vi "EXAMEND_13_02_25.vi"() -> ()   [LabVIEW 2025]
uses:
  <vilib>/numeric/Random Number (Range) I64.vi
  <vilib>/numeric/sub_Random U32.vi
panel:
  out "ESTADO DE LA SEÑAL":string
  out "ON/OFF":bool
  out "EN RANGO":bool
  out "VALOR PERILLA":dbl
  in  "Knob":dbl(knob) scale=0.0..100.0
  out "Valor Actual":dbl
  in  "stop":bool
  out "Waveform Chart":dynamicdata(graph)
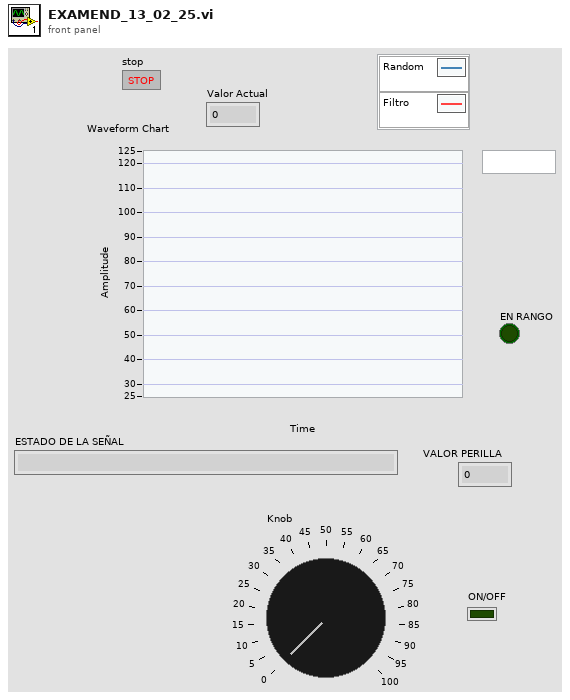
[diagram p1: front panel]
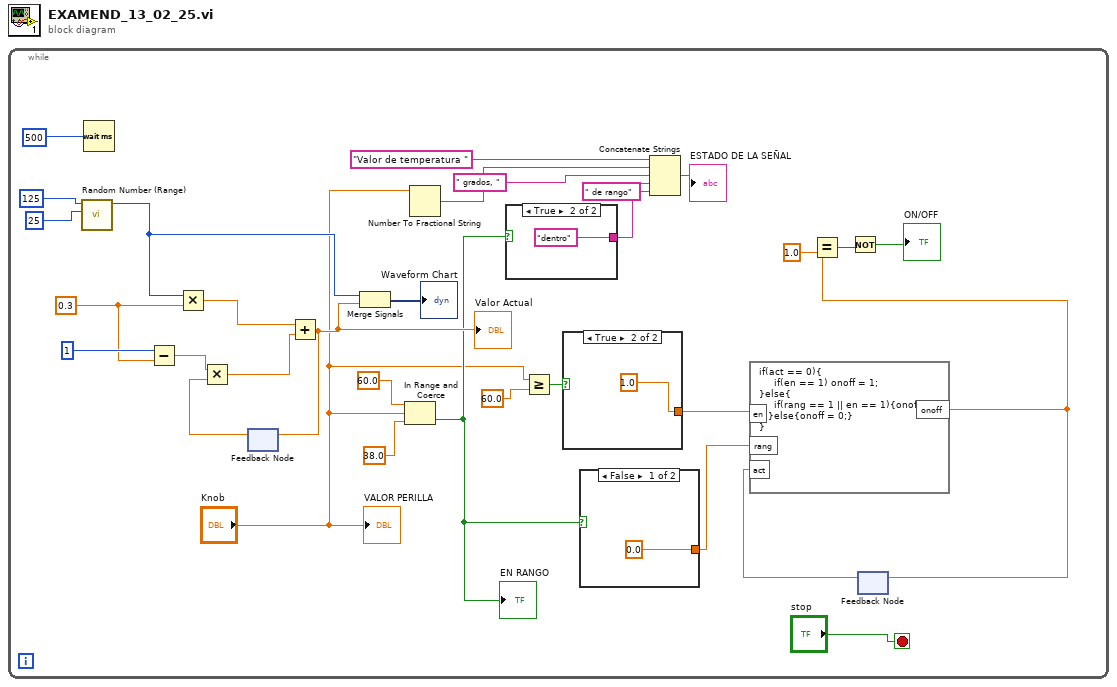
[diagram p0: block diagram]
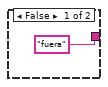
[diagram p2: hidden frame]
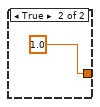
[diagram p3: hidden frame]
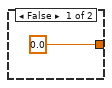
[diagram p4: hidden frame]
diagram:
  n1 = while {
    stop <- "stop" stop-if-true
    w29 = 0.3
    n2 = call-poly <vilib>:"Random Number (Range).vi"("lower bound (-100)"=25, "upper bound (100)"=125) -> ("number"=w21:i64)  [unwired: 9 in]
    n3 = Wait (ms)(milliseconds to wait=500) -> ()  [unwired: 1 out]
    n4 = Subtract(x=1, y=w29) -> (x-y=w28:dbl)
    n5 = Multiply(x=w21, y=w29) -> (x*y=w27:dbl)
    n6 = feedback #1() -> (w25:dbl)  [unwired: 1 in]
    n7 = Multiply(x=w28, y=w25) -> (x*y=w26:dbl)
    n8 = Add(x=w27, y=w26) -> (x+y=w10:dbl)
    "Valor Actual" <- w10
    n9 = feedback-in #1(w10) -> ()
    n10 = Merge Signals "Merge Signals"(w21, w10) -> (→"Waveform Chart":dynamicdata)
    n11 = In Range and Coerce(upper limit=60.0, x="Knob", lower limit=38.0) -> (In Range?=w6:bool)  [unwired: 1 out]
    "EN RANGO" <- w6
    n12 = Number To Fractional String(number="Knob") -> (F-format string=w9:string)  [unwired: 3 in]
    n13 = case shown="True" w6 {
      tunnel: ["fuera" ("string") "dentro" ("string")] -> w5
      frame False {
      }
      frame True {
      }
    }
    n14 = Greater Or Equal?(x="Knob", y=60.0) -> (x >= y?=w17:bool)
    n15 = case shown="True" w17 {
      tunnel: [0.0 1.0] -> w16
      frame False {
      }
      frame True {
      }
    }
    n16 = case shown="False" w6 {
      tunnel: [0.0 1.0] -> w15
      frame False {
      }
      frame True {
      }
    }
    n17 = Concatenate Strings("Valor de temperatura ", w9, " grados, " ("string"), w5, " de rango" ("string")) -> (→"ESTADO DE LA SEÑAL":string)
    n18 = feedback #2() -> (w14:dbl)  [unwired: 1 in]
    n19 = formula code="if(act == 0){\n     if(en == 1) onoff = 1;\n}else{\n     if(rang == 1 || en == 1){onoff = 1;}else{onoff = 0;}\n}"("en"=w16, "rang"=w15, "act"=w14) -> ("onoff"=w12:dbl)
    n20 = Equal?(x=w12, y=1.0) -> (x = y?=w2:bool)
    n21 = Not(x=w2) -> (.not. x?=→"ON/OFF":bool)
    n22 = feedback-in #2(w12) -> ()
    "VALOR PERILLA" <- "Knob"
  }
